vi "Setup Tab - Enable-Disable.vi"(5 "No.":refnum<vi>, 7 "MCListBox FHS Setup":refnum<vi>, 9 "[SRTRS][Config][ParameterSettings] - [userEditableProcedure]":bool, 10 "Disabled":T1(ring), 11 "Tab Setup":refnum<vi>) -> ()   [LabVIEW 2013]
panel:
  out "error out":errorcluster
  out "Main Label.Text":string[](array[string])
  out "ClassName":string[](array[string])
  out "Label.Text":string[](array[string])
  out "Page Label":string[](array[string])
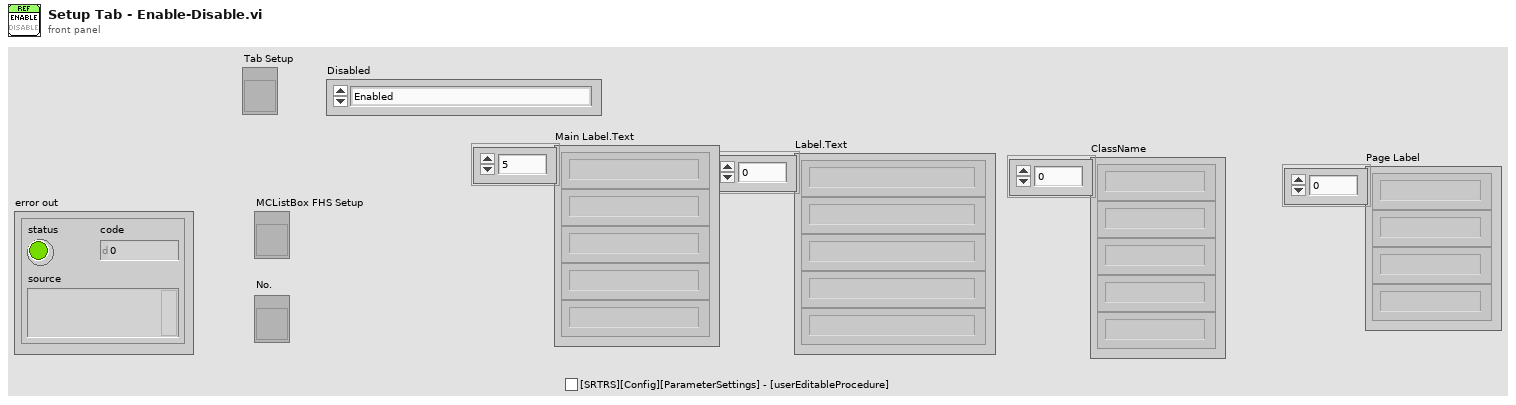
[diagram p1: front panel]
types:
  T1 = enum8{"Enabled", "Disabled", "Disabled and Grayed Out"}
  T2 = enum16{"Blank Cells Only", "Exisiting and Blank Cells"}
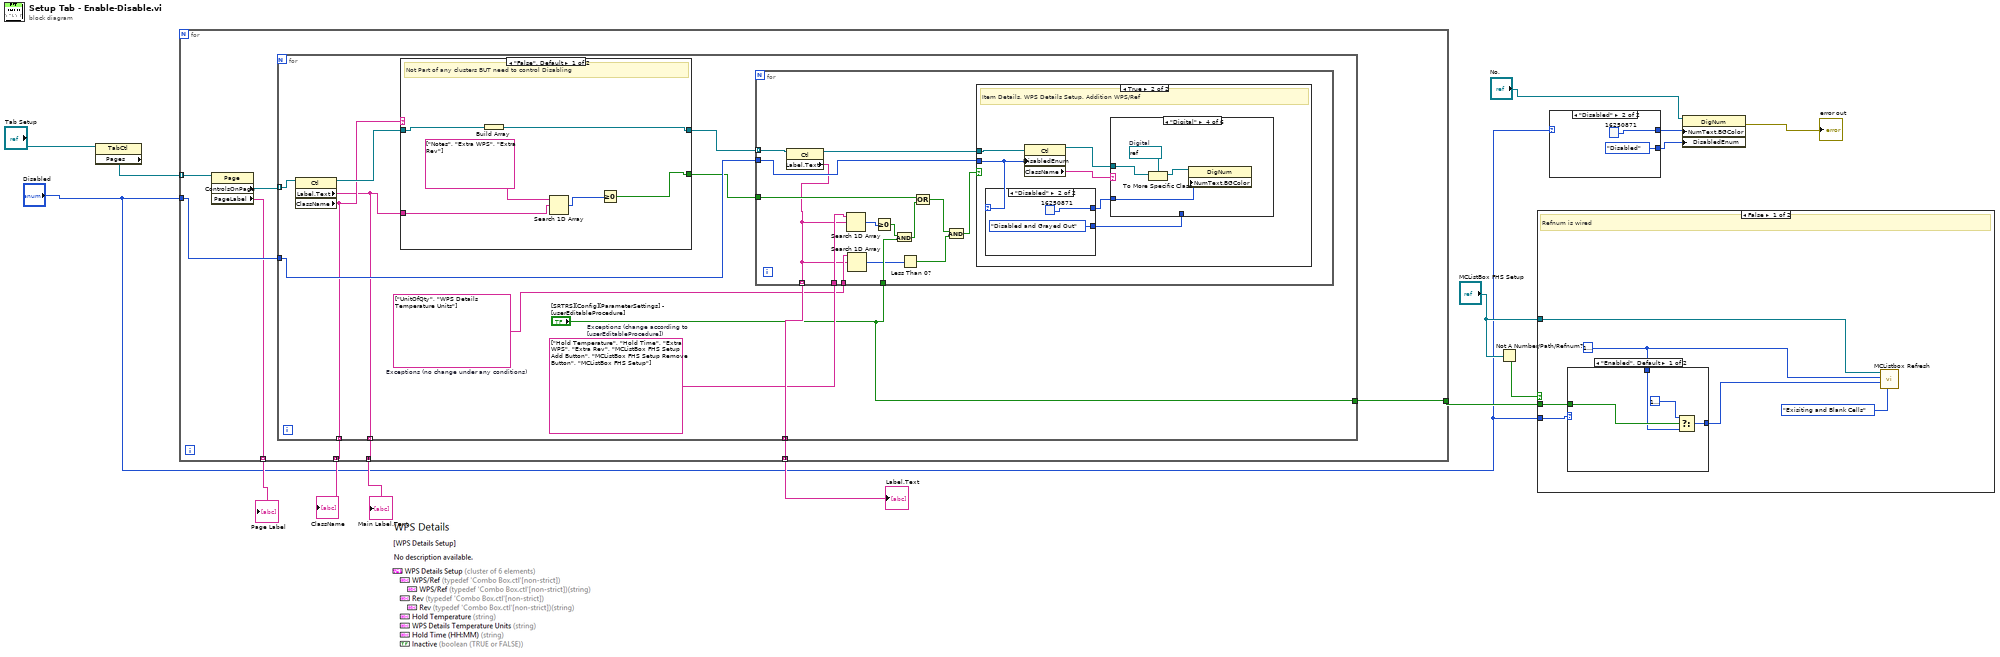
[diagram p0: block diagram]
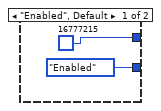
[diagram p2: hidden frame]
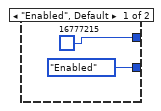
[diagram p6: hidden frame]
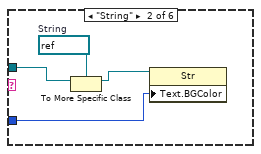
[diagram p8: hidden frame]
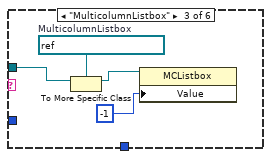
[diagram p9: hidden frame]
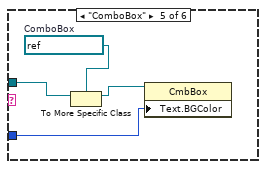
[diagram p10: hidden frame]
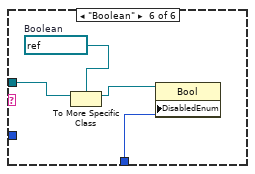
[diagram p11: hidden frame]
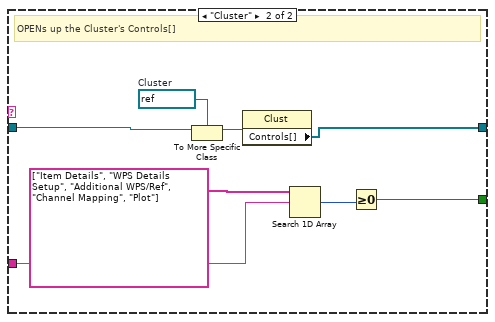
[diagram p12: hidden frame]
diagram:
  n1 = property class="TabCtl"(reference="Tab Setup") -> ("Pages"=w14:refnum<vi>[])  [unwired: 1 in, 2 out]
  n2 = for {
    tunnel: w14 -> [w22] mode=indexing
    tunnel: "Disabled" -> [w20]
    tunnel: [w19] -> w12 mode=indexing
    tunnel: [w18] -> w11 mode=concatenating
    tunnel: [w17] -> w10 mode=concatenating
    tunnel: [w16] -> w9 mode=concatenating
    tunnel: [w15] -> w7
    n3 = property class="Page"(reference=w22) -> ("ControlsOnPage"=w21:refnum<vi>[], "PageLabel"=w19:string)  [unwired: 1 in, 2 out]
    n4 = for {
      tunnel: w21 -> [w33] mode=indexing
      tunnel: w20 -> [w31]
      tunnel: [w28] -> w18 mode=indexing
      tunnel: [w29] -> w17 mode=concatenating
      tunnel: [w25] -> w16 mode=indexing
      tunnel: ["[SRTRS][Config][ParameterSettings] - [userEditableProcedure]"] -> w15
      w24 = string[] ["UnitOfQty", "WPS Details Temperature Units"]  # Exceptions (no change under any conditions)
      w27 = string[] ["Hold Temperature", "Hold Time", "Extra WPS", "Extra Rev", "MCListBox FHS Setup Add Button", "MCListBox FHS Setup Remove Button", "MCListBox FHS Setup"]  # Exceptions (change according to [userEditableProcedure])
      n5 = property class="Ctl"(reference=w33) -> (reference out=w32:refnum<vi>, "Label.Text"=w25:string, "ClassName"=w28:string)  [unwired: 1 in, 1 out]
      n6 = case shown="\"False\", Default" w28 {
        tunnel: w32 -> [w84 w92]
        tunnel: [w83 w86] -> w30
        tunnel: w25 -> [w82 w89]
        tunnel: [w79 w85] -> w26
        frame "False", Default {
          # "Not Part of any clusters BUT need to control Disabling"
          n7 = Build Array(w84) -> (w83:refnum<vi>[])
          n8 = Search 1D Array(1D array=string[] ["Notes", "Extra WPS", "Extra Rev"], element=w82) -> (index of element=w80:i32)  [unwired: 1 in]
          n9 = Greater Or Equal To 0?(x=w80) -> (x >= 0?=w79:bool)
        }
        frame "Cluster" {
          w87 = refnum<vi> refnum  # Cluster
          # "OPENs up the Cluster's Controls[]"
          n10 = To More Specific Class(target class=w87, reference=w92) -> (specific class reference=w91:refnum<vi>)  [unwired: 1 in, 1 out]
          n11 = property class="Clust"(reference=w91) -> ("Controls[]"=w86:refnum<vi>[])  [unwired: 1 in, 2 out]
          n12 = Search 1D Array(1D array=string[] ["Item Details", "WPS Details Setup", "Additional WPS/Ref", "Channel Mapping", "Plot"], element=w89) -> (index of element=w88:i32)  [unwired: 1 in]
          n13 = Greater Or Equal To 0?(x=w88) -> (x >= 0?=w85:bool)
        }
      }
      n14 = for {
        tunnel: w31 -> [w48]
        tunnel: w30 -> [w47] mode=indexing
        tunnel: [w38] -> w29 mode=indexing
        tunnel: w27 -> [w45]
        tunnel: "[SRTRS][Config][ParameterSettings] - [userEditableProcedure]" -> [w42]
        tunnel: w26 -> [w40]
        tunnel: w24 -> [w39]
        n15 = property class="Ctl"(reference=w47) -> (reference out=w46:refnum<vi>, "Label.Text"=w38:string)  [unwired: 1 in, 1 out]
        n16 = Search 1D Array(1D array=w45, element=w38) -> (index of element=w44:i32)  [unwired: 1 in]
        n17 = Search 1D Array(1D array=w39, element=w38) -> (index of element=w36:i32)  [unwired: 1 in]
        n18 = Greater Or Equal To 0?(x=w44) -> (x >= 0?=w43:bool)
        n19 = And(x=w43, y=w42) -> (x .and. y?=w41:bool)
        n20 = Less Than 0?(x=w36) -> (x < 0?=w35:bool)
        n21 = Or(x=w40, y=w41) -> (x .or. y?=w37:bool)
        n22 = And(x=w37, y=w35) -> (x .and. y?=w34:bool)
        n23 = case shown="True" w34 {
          tunnel: w48 -> [_ w54]
          tunnel: w46 -> [_ w53]
          frame False {
          }
          frame True {
            # "Item Details, WPS Details Setup, Addition WPS/Ref"
            n24 = case shown="\"Disabled\"" w54 {
              tunnel: [u32 16777215 u32 16250871] -> w50
              tunnel: [T1."Enabled" ("Disabled") T1."Disabled and Grayed Out" ("Disabled")] -> w49
              frame "Enabled", Default {
              }
              frame "Disabled" {
              }
            }
            n25 = property class="Ctl"(reference=w53, "DisabledEnum"=w54) -> (reference out=w51:refnum<vi>, "ClassName"=w52:string)  [unwired: 1 in, 1 out]
            n26 = case shown="\"Digital\"" w52 {
              tunnel: w51 -> [_ w62 w66 w70 w74 w78]
              tunnel: w50 -> [_ w59 _ w67 w71 _]
              tunnel: w49 -> [_ _ _ _ _ w75]
              frame "False", Default {
              }
              frame "String" {
                w61 = refnum<vi> refnum  # String
                n27 = To More Specific Class(target class=w61, reference=w62) -> (specific class reference=w60:refnum<vi>)  [unwired: 1 in, 1 out]
                n28 = property class="Str"(reference=w60, "Text.BGColor"=w59) -> ()  [unwired: 1 in, 2 out]
              }
              frame "MulticolumnListbox" {
                w65 = refnum<vi> refnum  # MulticolumnListbox
                n29 = To More Specific Class(target class=w65, reference=w66) -> (specific class reference=w64:refnum<vi>)  [unwired: 1 in, 1 out]
                n30 = property class="MCListbox"(reference=w64, "Value"=-1) -> ()  [unwired: 1 in, 2 out]
              }
              frame "Digital" {
                w69 = refnum<vi> refnum  # Digital
                n31 = To More Specific Class(target class=w69, reference=w70) -> (specific class reference=w68:refnum<vi>)  [unwired: 1 in, 1 out]
                n32 = property class="DigNum"(reference=w68, "NumText.BGColor"=w67) -> ()  [unwired: 1 in, 2 out]
              }
              frame "ComboBox" {
                w72 = refnum<vi> refnum  # ComboBox
                n33 = To More Specific Class(target class=w72, reference=w74) -> (specific class reference=w73:refnum<vi>)  [unwired: 1 in, 1 out]
                n34 = property class="CmbBox"(reference=w73, "Text.BGColor"=w71) -> ()  [unwired: 1 in, 2 out]
              }
              frame "Boolean" {
                w76 = refnum<vi> refnum  # Boolean
                n35 = To More Specific Class(target class=w76, reference=w78) -> (specific class reference=w77:refnum<vi>)  [unwired: 1 in, 1 out]
                n36 = property class="Bool"(reference=w77, "DisabledEnum"=w75) -> ()  [unwired: 1 in, 2 out]
              }
            }
          }
        }
      }
    }
  }
  "Page Label" <- w12
  "Label.Text" <- w10
  "ClassName" <- w11
  "Main Label.Text" <- w9
  n37 = Not A Number/Path/Refnum?(number/path/refnum="MCListBox FHS Setup") -> (NaN/Path/Refnum?=w8:bool)
  n38 = case shown="False" w8 {
    tunnel: "MCListBox FHS Setup" -> [w97 _]
    tunnel: "Disabled" -> [w96 _]
    tunnel: w7 -> [w95 _]
    frame False {
      w94 = u32 16777238 ("color of Blank cells")
      # "Refnum is wired"
      n39 = case shown="\"Enabled\", Default" w96 {
        tunnel: w95 -> [w102 _]
        tunnel: w94 -> [w100 w103]
        tunnel: [w99 w103] -> w93
        frame "Enabled", Default {
          n40 = Select(t=u32 16777225 ("color of New Cells"), s=w102, f=w100) -> (s? t:f=w99:u32)
        }
        frame "Disabled" {
        }
      }
      n41 = call "MCListbox Refresh.vi"("Which Cells"=T2."Exisiting and Blank Cells", "color of New Cells"=w93, "color of Blank cells"=w94, "MulticolumnListbox in"=w97) -> ()  [unwired: 6 in, 2 out]
    }
    frame True {
      # "Not a Refnum"
    }
  }
  n42 = case shown="\"Disabled\"" "Disabled" {
    tunnel: [u32 16777215 u32 16250871] -> w1
    tunnel: [T1."Enabled" ("Disabled") T1."Disabled" ("Disabled")] -> w2
    frame "Enabled", Default {
    }
    frame "Disabled" {
    }
  }
  n43 = property class="DigNum"(reference="No.", "NumText.BGColor"=w1, "DisabledEnum"=w2) -> (error out=→"error out":errorcluster)  [unwired: 1 in, 1 out]
